vi "_Set LED.vi"(3 "LED States":T1) -> ()   [LabVIEW 2012]
uses:
  Type/_LED States.ctl
  <vilib>/rvi/DataTransferAndStorage/Container/Common/niFpgaContainerGetUniqueNameForEmu.vi
  <vilib>/rvi/Memory/Memory_Emulation/niFpgaMemoryEmulationCacheClearOnFirstRun.vi
  <vilib>/rvi/Memory/Memory_Emulation/nirvimemoryEmulationManagerCache_MakeExclusive.vi
  <vilib>/rvi/Memory/Memory_Emulation/niFpgaMemoryEmulationValidateCache.vi
  <vilib>/rvi/Memory/Memory_Emulation/nirvimemoryEmulationManagerCache_ReleaseExclusive.vi
  <vilib>/rvi/Memory/Memory_Emulation/nirvimemoryEmulationManagerCache_InsertValue.vi
  <vilib>/Utility/error.llb/Clear Errors.vi
  <vilib>/rvi/Emulation/niFpgaSctlEmulationGetInTimedLoop.vi
  <vilib>/rvi/Memory/Memory_Emulation/nirvimemoryEmulationManagerCache_GetValue.vi
  <vilib>/rvi/Memory/Memory_Emulation/nirvimemoryEmulationManagerCache_SetValue.vi
  <vilib>/rvi/Emulation/niFpgaSctlEmulationResourceMgr.vi
  <vilib>/rvi/DataTransferAndStorage/Container/XNode/niFpgaContainer.xnode
  <vilib>/rvi/Memory/Memory_Emulation/nirvimemoryEmulation.vi
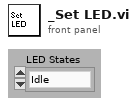
[diagram p1: front panel]
types:
  T1 = typedef "_LED States.ctl" = enum8{"Idle", "Solid B", "Solid R", "Solid P", "Off B", "Off R", "Off P", "Off BRP", "Off RP", "Flash R&P", "Flash P"}
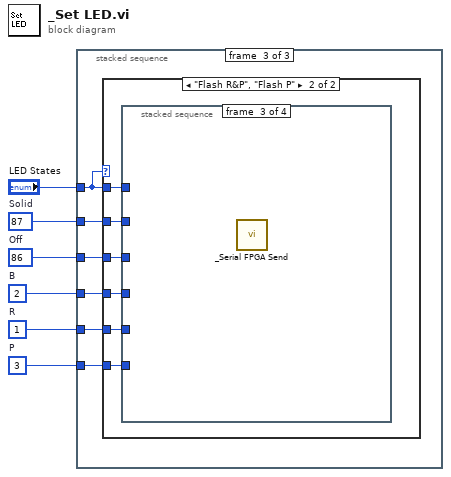
[diagram p0: block diagram]
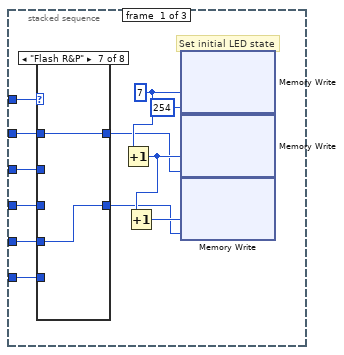
[diagram p2: hidden frame]
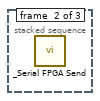
[diagram p10: hidden frame]
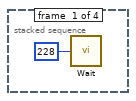
[diagram p12: hidden frame]
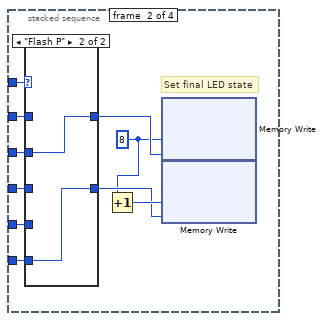
[diagram p13: hidden frame]
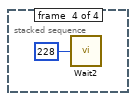
[diagram p15: hidden frame]
diagram:
  w1 = u8 3  # P
  w2 = u8 1  # R
  w3 = u8 2  # B
  w4 = u8 86  # Off
  w5 = u8 87  # Solid
  n1 = stacked-sequence {
    tunnel: "LED States" -> [w14 _ w35]
    tunnel: w5 -> [w13 _ w40]
    tunnel: w4 -> [w12 _ w39]
    tunnel: w3 -> [w11 _ w38]
    tunnel: w2 -> [w10 _ w37]
    tunnel: w1 -> [w9 _ w36]
    frame #0 {
      w16 = u8 7 ("Address")
      # "Set initial LED state"
      n2 = case shown="\"Flash R&P\"" w14 {
        tunnel: w13 -> [w19 w22 w24 _ _ _ w32 w34]
        tunnel: w12 -> [_ _ _ w26 w28 w30 _ _]
        tunnel: w11 -> [_ w21 _ w25 _ _ _ _]
        tunnel: w10 -> [w20 _ _ _ w27 _ w31 _]
        tunnel: w9 -> [_ _ w23 _ _ w29 _ w33]
        tunnel: [w19 w22 w24 w26 w28 w30 w32 w34] -> w8
        tunnel: [w20 w21 w23 w25 w27 w29 w31 w33] -> w7
        frame "Idle", "Solid R", Default {
        }
        frame "Solid B" {
        }
        frame "Solid P" {
        }
        frame "Off B", "Off BRP" {
        }
        frame "Off R", "Off RP" {
        }
        frame "Off P" {
        }
        frame "Flash R&P" {
        }
        frame "Flash P" {
        }
      }
      n3 = Increment(x=w16) -> (x+1=w17:u8)
      n4 = Increment(x=w17) -> (x+1=w18:u8)
      n5 = xnode ("Memory Write")("Address"=w16, "Data"=u8 254) -> ()  [unwired: 1 in, 1 out]
      n6 = xnode ("Memory Write")("Address"=w17, "Data"=w8) -> ()  [unwired: 1 in, 1 out]
      n7 = xnode ("Memory Write")("Address"=w18, "Data"=w7) -> ()  [unwired: 1 in, 1 out]
    }
    frame #1 {
      n8 = call "_Serial FPGA Send.vi"() -> ()  [unwired: 1 in]
    }
    frame #2 {
      n9 = case shown="\"Flash R&P\", \"Flash P\"" w35 {
        tunnel: w35 -> [_ w46]
        tunnel: w40 -> [_ w45]
        tunnel: w39 -> [_ w44]
        tunnel: w38 -> [_ w43]
        tunnel: w37 -> [_ w42]
        tunnel: w36 -> [_ w41]
        frame "Idle", Default {
        }
        frame "Flash R&P", "Flash P" {
          n10 = stacked-sequence {
            tunnel: w46 -> [_ w56 _ _]
            tunnel: w45 -> [_ w55 _ _]
            tunnel: w44 -> [_ w54 _ _]
            tunnel: w43 -> [_ w53 _ _]
            tunnel: w42 -> [_ w52 _ _]
            tunnel: w41 -> [_ w51 _ _]
            frame #0 {
              n11 = call "Wait"("Count(mSec)"=u8 228) -> ()  [unwired: 1 out]
            }
            frame #1 {
              w48 = u8 8 ("Address")
              # "Set final LED state"
              n12 = case shown="\"Flash P\"" w56 {
                tunnel: w55 -> [_ _]
                tunnel: w54 -> [w58 w60]
                tunnel: w53 -> [_ _]
                tunnel: w52 -> [w59 _]
                tunnel: w51 -> [_ w61]
                tunnel: [w58 w60] -> w50
                tunnel: [w59 w61] -> w49
                frame "Flash R&P", Default {
                }
                frame "Flash P" {
                }
              }
              n13 = Increment(x=w48) -> (x+1=w57:u8)
              n14 = xnode ("Memory Write")("Address"=w48, "Data"=w50) -> ()  [unwired: 1 in, 1 out]
              n15 = xnode ("Memory Write")("Address"=w57, "Data"=w49) -> ()  [unwired: 1 in, 1 out]
            }
            frame #2 {
              n16 = call "_Serial FPGA Send.vi"() -> ()  [unwired: 1 in]
            }
            frame #3 {
              n17 = call "Wait2"("Count(mSec)"=u8 228) -> ()  [unwired: 1 out]
            }
          }
        }
      }
    }
  }
